vi "initZ.vi"(2 "zIdx":i32=1, 3 "System no.":i32=2 min=1 step=1) -> (0 "zLim":dbl, 1 "zPos":dbl)   [LabVIEW 2015]
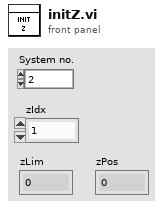
[diagram p1: front panel]
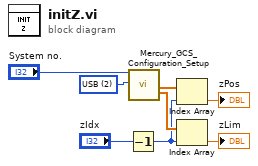
[diagram p0: block diagram]
diagram:
  w7 = u16 2 items=["RS232", "RS232 DaisyChain", "USB", "USB_DaisyChain"] ("Interface")
  n1 = Decrement(x="zIdx") -> (x-1=w1:i32)
  n2 = call "Mercury_GCS_Configuration_Setup.vi"("System no."="System no.", "Interface"=w7) -> ("Position"=w5:dbl[], "+/- movement\nrange"=w6:dbl[])  [unwired: 11 in, 5 out]
  n3 = Index Array(array=w5, index=w1) -> (element=→"zPos":dbl)
  n4 = Index Array(array=w6, index=w1) -> (element=→"zLim":dbl)
